vi "ziExample1-PollDemod.vi"(0 "Address":string="DEV", 1 "stop":bool) -> (20 "Selected Device":string)   [LabVIEW 2016]
doc: "Control a Zurich instrument device via the LabOne Labview API. \nRequirements: Zurich Instruments MFLI, HF2 or UHFLI \nThis example polls demod data for a given time from the instrument.\n\n© Zurich Instruments AG, www.zhinst.com"
uses:
  <instrlib>/Zurich Instruments LabOne/Public/Utility/ziTicksToS_vector.vi
  <instrlib>/Zurich Instruments LabOne/Zurich Instruments LabOne.lvlib
panel:
  in  "Subscribe Path Array":string[](array[string])=["demods/0/sample"]
  out "Error Out":errorcluster
  out "XY Graph":cluster{dbl[], "X (Vrms)":dbl[]}[](graph)
  in  "time":dbl=1.0 caption="recording time [s]"
  # "ziExample-PollDemod.vi\nRequirements: HF2, UHFLI or MFLI\nsee block diagram for VI description"
  # "Tested Instruments:\n- MFLI\n- HF2LI\n- UHFLI"
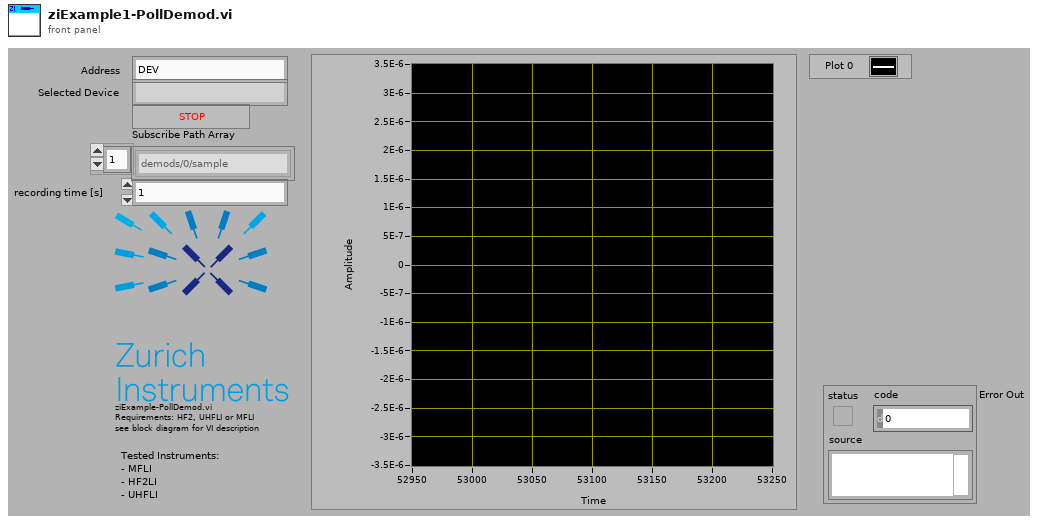
[diagram p1: front panel]
types:
  T1 = typedef "Zurich Instruments LabOne.lvlib/ziTypeHandle.ctl" = cluster{"handleValid":bool, "Conn":u64, "Path Prefix":string, "Handle":u64, "Connected":bool, "Clockbase(s)":dbl}
  T2 = typedef "Zurich Instruments LabOne.lvlib/ziTypeDemodSampleEx.ctl" = cluster{"Timestamps (ticks)":u64[], "X (Vrms)":dbl[], "Y (Vrms)":dbl[], "Osc Phase (rad)":dbl[], "Freq (Hz)":dbl[], "DIO":u32[], "Aux In 0 (V)":dbl[], "Aux In 1 (V)":dbl[], "Trigger":u32[]}
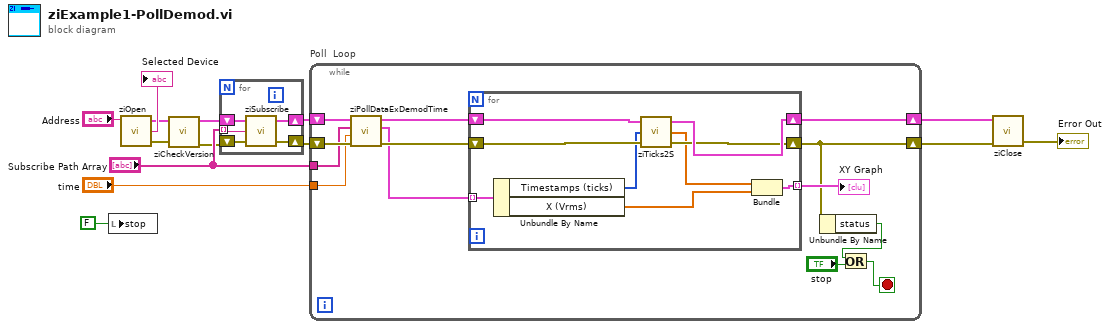
[diagram p0: block diagram]
diagram:
  n1 = local write "stop"(FALSE ("stop")) -> ()
  n2 = call <instrlib>:"ziOpen.vi"("Address"="Address") -> ("Error Out"=w3:errorcluster, "Selected Device"=→"Selected Device":string, "HandleOut"=w4:T1)  [unwired: 1 in, 2 out]
  n3 = call <instrlib>:"ziCheckVersion.vi"("Handle In"=w4, "Error In"=w3) -> ("Handle Out"=w1:T1, "Error Out"=w2:errorcluster)  [unwired: 11 in, 1 out]
  n4 = for {
    tunnel: "Subscribe Path Array" -> [w15] mode=indexing
    shift-right: [w17] -> w9
    shift-left: w2 -> [w18]
    shift-right: [w16] -> w8
    shift-left: w1 -> [w19]
    n5 = call <instrlib>:"ziSubscribe.vi"("error in"=w18, "Path ()"=w15, "Handle In"=w19) -> ("error out"=w17:errorcluster, "Handle Out"=w16:T1)  [unwired: 1 in]
  }
  n6 = while "Poll  Loop" {
    shift-right: [w27] -> w14
    shift-left: w8 -> [w31]
    shift-right: [w23] -> w11
    shift-left: w9 -> [w32]
    tunnel: "Subscribe Path Array" -> [w30]
    tunnel: "time" -> [w25]
    stop <- w20 stop-if-true
    n7 = call <instrlib>:"ziPollDataExDemodTime.vi"("error in"=w32, "recording time (1) [s]"=w25, "SubscribepathArray"=w30, "Handle In"=w31) -> ("error out"=w29:errorcluster, "Demod Sample Out"=w26:T2[], "Handle Out"=w28:T1)  [unwired: 5 in]
    n8 = for {
      tunnel: w26 -> [w37] mode=indexing
      shift-right: [w38] -> w23
      shift-left: w29 -> [w41]
      shift-right: [w39] -> w27
      shift-left: w28 -> [w40]
      tunnel: [w35] -> w24 mode=indexing
      n9 = Unbundle By Name(w37) -> ("Timestamps (ticks)"=w36:u64[], "X (Vrms)"=w34:dbl[])
      n10 = call-poly <instrlib>:"ziTicks2S.vi"("Error In"=w41, "Timestamp (ticks)"=w36, "Handle In"=w40) -> ("Error Out"=w38:errorcluster, "Timestamp(s)"=w33:dbl[], "Handle Out"=w39:T1)
      n11 = Bundle("Timestamp(s)"=w33, "X (Vrms)"=w34) -> (w35:cluster{"Timestamp(s)":dbl[], "X (Vrms)":dbl[]})  [unwired: 1 in]
    }
    "XY Graph" <- w24
    n12 = Unbundle By Name(w23) -> ("status"=w21:bool)
    n13 = Or(x=w21, y="stop") -> (x .or. y?=w20:bool)
  }
  n14 = call <instrlib>:"ziClose.vi"("Error In"=w11, "Handle In"=w14) -> ("Error Out"=→"Error Out":errorcluster)  [unwired: 3 out]
